vi "Motor Joystick Increment.vi"() -> ()   [LabVIEW 2012]
uses:
  <vilib>/Rock Robotics/SystemInterfaces/DIO/FPGA_DIOPWMChannel.ctl
  <vilib>/Rock Robotics/WPI/Joystick/WPI_JoystickDeviceEnum.ctl
  <vilib>/Rock Robotics/WPI/MotorControl/WPI_MotorControlOpen Talon.vi
panel:
  in  "On/Off":bool
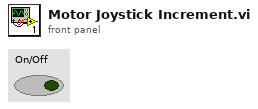
[diagram p1: front panel]
types:
  T1 = typedef "WPI_JoystickDeviceEnum.ctl" = enum16{"USB 1", "USB 2", "USB 3", "USB 4", "Kinect 1", "Kinect 2"}
  T2 = typedef "FPGA_DIOPWMChannel.ctl" = enum8{"PWM 1", "PWM 2", "PWM 3", "PWM 4", "PWM 5", "PWM 6", "PWM 7", "PWM 8", "PWM 9", "PWM 10", "Invalid"}
  T3 = typedef "WPI_MotorControlDeviceRef.ctl" = cluster{"DeviceStatus":errorcluster, "Type":enum16{"PWM", "CAN"}, "PWM":cluster{"Digital Module":T4, "PWM Channel":T2, "DeadBand":T5}, "CAN":cluster{"Device Number":u8, "Control Mode":T6, "Semaphore":T7, "Max Vout":dbl}, "Invert":bool, "TransformRef":T8, "InvTransformRef":T8}
  T4 = typedef "FPGA_TypedefDigitalModule.ctl" = enum16{"Digital Module 1", "Digital Module 2"}
  T5 = typedef "WPI_PWMDeadband.ctl" = cluster{"Name":string, "maxPositivePwm":i32, "minPositivePwm":i32, "centerPwm":i32, "maxNegativePwm":i32, "minNegativePwm":i32, "angularRange":u16}
  T6 = typedef "WPI_CANJaguar_ControlMode.ctl" = enum8{"Percent VBus", "Current", "Speed", "Position", "Voltage"}
  T7 = typedef "Semaphore RefNum" = refnum<k1>
  T8 = typedef "WPI_PWMTransform_ConPane.ctl" = refnum<vi>
  T9 = typedef "WPI_JoystickDevRef.ctl" = cluster{"Device":T1}
  T10 = cluster{"axis 1 (x)":dbl, "axis 2 (y)":dbl, "axis 3 (throttle)":dbl, "axis 4":dbl, "axis 5":dbl, "axis 6":dbl}
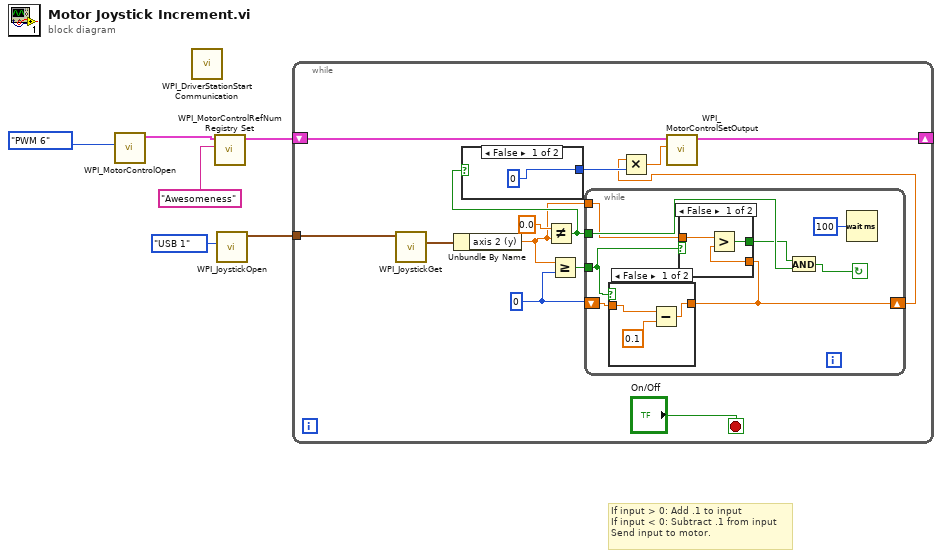
[diagram p0: block diagram]
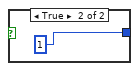
[diagram p2: hidden frame]
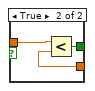
[diagram p3: hidden frame]
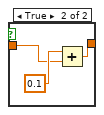
[diagram p4: hidden frame]
diagram:
  # "If input > 0: Add .1 to input\nIf input < 0: Subtract .1 from input\nSend input to motor."
  n1 = call-poly <vilib>:"WPI_MotorControlOpen.vi"("PWM Channel"=FPGA_DIOPWMChannel."PWM 6") -> ("MotorControlDeviceRef"=w3:T3)  [unwired: 9 in, 1 out]
  n2 = call <vilib>:"WPI_DriverStationStart Communication.vi"() -> ()  [unwired: 12 in]
  n3 = call <vilib>:"WPI_MotorControlRefNum Registry Set.vi"("refnum name"="Awesomeness", "MotorControlDevRef"=w3) -> ("MotorControlDevRef"=w1:T3)  [unwired: 8 in, 1 out]
  n4 = call <vilib>:"WPI_JoystickOpen.vi"("JoystickDevice"=WPI_JoystickDeviceEnum."USB 1") -> ("JoystickDevRef"=w4:T9)  [unwired: 10 in]
  n5 = while {
    tunnel: w4 -> [w19]
    shift-right: [w15] -> _
    shift-left: w1 -> [w16]
    stop <- "On/Off" stop-if-true
    w8 = 0
    n6 = call <vilib>:"WPI_JoystickGet.vi"("JoystickDevRef"=w19) -> ("Axes"=w18:T10)  [unwired: 4 in, 2 out]
    n7 = Unbundle By Name(w18) -> ("axis 2 (y)"=w9:dbl)
    n8 = Not Equal?(x=0.0, y=w9) -> (x != y?=w13:bool)
    n9 = case shown="False" w13 {
      tunnel: [0 1] -> w12
      frame False {
      }
      frame True {
      }
    }
    n10 = Greater Or Equal?(x=w9, y=w8) -> (x >= y?=w7:bool)
    n11 = while {
      tunnel: w13 -> [w27]
      tunnel: w9 -> [w24]
      shift-right: [w23] -> w11
      shift-left: w8 -> [w29]
      tunnel: w7 -> [w25]
      stop <- w26 continue-if-true
      n12 = case shown="False" w25 {
        tunnel: w29 -> [w37 w40]
        tunnel: [w38 w39] -> w23
        frame False {
          n13 = Subtract(x=w37, y=0.1) -> (x-y=w38:dbl)
        }
        frame True {
          n14 = Add(x=0.1, y=w40) -> (x+y=w39:dbl)
        }
      }
      n15 = case shown="False" w25 {
        tunnel: w24 -> [w31 w35]
        tunnel: w23 -> [w30 w34]
        tunnel: [w32 w33] -> w22
        frame False {
          n16 = Greater?(x=w31, y=w30) -> (0:w32:bool)
        }
        frame True {
          n17 = Less?(x=w35, y=w34) -> (x < y?=w33:bool)
        }
      }
      n18 = And(x=w22, y=w27) -> (x .and. y?=w26:bool)
      n19 = Wait (ms)(milliseconds to wait=u32 100) -> ()  [unwired: 1 out]
    }
    n20 = Multiply(x=w11, y=w12) -> (x*y=w10:dbl)
    n21 = call <vilib>:"WPI_MotorControlSetOutput.vi"("Output"=w10, "MotorControlDevRef"=w16) -> ("MotorControlDevRef"=w15:T3)  [unwired: 7 in, 2 out]
  }
